vi "FGV_SyncData.vi"(10 "Data In":T1[](array[typedef]), 11 "Mode":enum16{"Get", "Set", "Init"}(ring)) -> (2 "Data out":T1[](array[typedef]))   [LabVIEW 2016]
uses:
  DAQ_ReadBlock.ctl
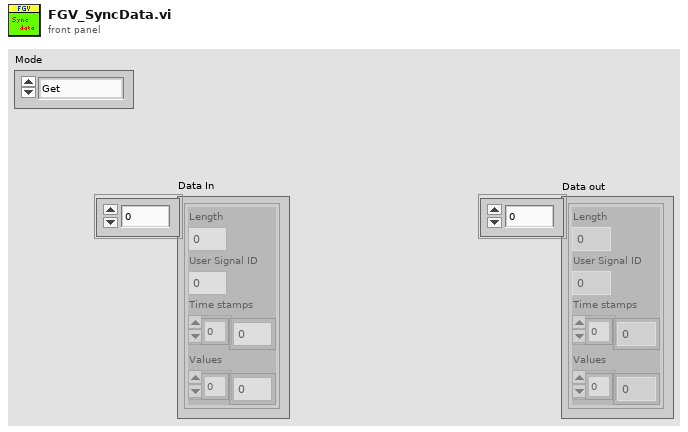
[diagram p1: front panel]
types:
  T1 = typedef "DAQ_ReadBlock.ctl" = cluster{"Length":i32, "User Signal ID":i32, "Time stamps":dbl[], "Values":dbl[]}
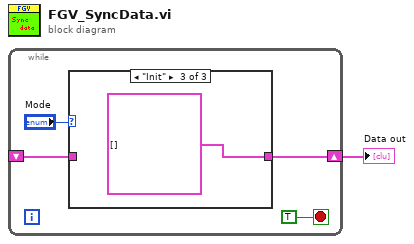
[diagram p0: block diagram]
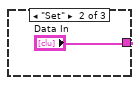
[diagram p3: hidden frame]
diagram:
  n1 = while {
    shift-right: [w3] -> w1
    shift-left: _ -> [w4]
    stop <- TRUE stop-if-true
    n2 = case shown="\"Init\"" "Mode" {
      tunnel: w4 -> [w6 _ _]
      tunnel: [w6 "Data In" T1[] []] -> w3
      frame "Get", Default {
      }
      frame "Set" {
      }
      frame "Init" {
      }
    }
  }
  "Data out" <- w1
